vi "createPlatformDataV2.vi"() -> (3 "digital waveform":bool[](array[boolean]))   [LabVIEW 2017]
panel:
  in  "Platform 61":bool
  in  "Platform 60":bool
  in  "Platform 59":bool
  in  "Platform 58":bool
  in  "Platform 57":bool
  in  "Platform 56":bool
  in  "Platform 55":bool
  in  "Platform 54":bool
  in  "Platform 53":bool
  in  "Platform 52":bool
  in  "Platform 51":bool
  in  "Platform 50":bool
  in  "Platform 49":bool
  in  "Platform 48":bool
  in  "Platform 47":bool
  in  "Platform 46":bool
  in  "Platform 45":bool
  in  "Platform 44":bool
  in  "Platform 43":bool
  in  "Platform 42":bool
  in  "Platform 41":bool
  in  "Platform 40":bool
  in  "Platform 39":bool
  in  "Platform 38":bool
  in  "Platform 37":bool
  in  "Platform 36":bool
  in  "Platform 35":bool
  in  "Platform 34":bool
  in  "Platform 33":bool
  in  "Platform 32":bool
  in  "Platform 31":bool
  in  "Platform 30":bool
  in  "Platform 29":bool
  in  "Platform 28":bool
  in  "Platform 27":bool
  in  "Platform 26":bool
  in  "Platform 25":bool
  in  "Platform 24":bool
  in  "Platform 23":bool
  in  "Platform 22":bool
  in  "Platform 21":bool
  in  "Platform 20":bool
  in  "Platform 19":bool
  in  "Platform 18":bool
  in  "Platform 17":bool
  in  "Platform 16":bool
  in  "Platform 15":bool
  in  "Platform 14":bool
  in  "Platform 13":bool
  in  "Platform 12":bool
  in  "Platform 11":bool
  in  "Platform 10":bool
  in  "Platform 9":bool
  in  "Platform 8":bool
  in  "Platform 7":bool
  in  "Platform 6":bool
  in  "Platform 5":bool
  in  "Platform 4":bool
  in  "Platform 3":bool
  in  "Platform 2":bool
  in  "Platform 1":bool
  in  "Select?":bool
  in  "Platform 61":bool
  in  "Platform 60":bool
  in  "Platform 59":bool
  in  "Platform 58":bool
  in  "Platform 57":bool
  in  "Platform 56":bool
  in  "Platform 55":bool
  in  "Platform 54":bool
  in  "Platform 53":bool
  in  "Platform 52":bool
  in  "Platform 51":bool
  in  "Platform 50":bool
  in  "Platform 49":bool
  in  "Platform 48":bool
  in  "Platform 47":bool
  in  "Platform 46":bool
  in  "Platform 45":bool
  in  "Platform 44":bool
  in  "Platform 43":bool
  in  "Platform 42":bool
  in  "Platform 41":bool
  in  "Platform 40":bool
  in  "Platform 39":bool
  in  "Platform 38":bool
  in  "Platform 37":bool
  in  "Platform 36":bool
  in  "Platform 35":bool
  in  "Platform 34":bool
  in  "Platform 33":bool
  in  "Platform 32":bool
  in  "Platform 31":bool
  in  "Platform 30":bool
  in  "Platform 29":bool
  in  "Platform 28":bool
  in  "Platform 27":bool
  in  "Platform 26":bool
  in  "Platform 25":bool
  in  "Platform 24":bool
  in  "Platform 23":bool
  in  "Platform 22":bool
  in  "Platform 21":bool
  in  "Platform 20":bool
  in  "Platform 19":bool
  in  "Platform 18":bool
  in  "Platform 17":bool
  in  "Platform 16":bool
  in  "Platform 15":bool
  in  "Platform 14":bool
  in  "Platform 13":bool
  in  "Platform 12":bool
  in  "Platform 11":bool
  in  "Platform 10":bool
  in  "Platform 9":bool
  in  "Platform 8":bool
  in  "Platform 7":bool
  in  "Platform 6":bool
  in  "Platform 5":bool
  in  "Platform 4":bool
  in  "Platform 3":bool
  in  "Platform 2":bool
  in  "Platform 1":bool
  # "Platforms up"
  # "Platforms down"
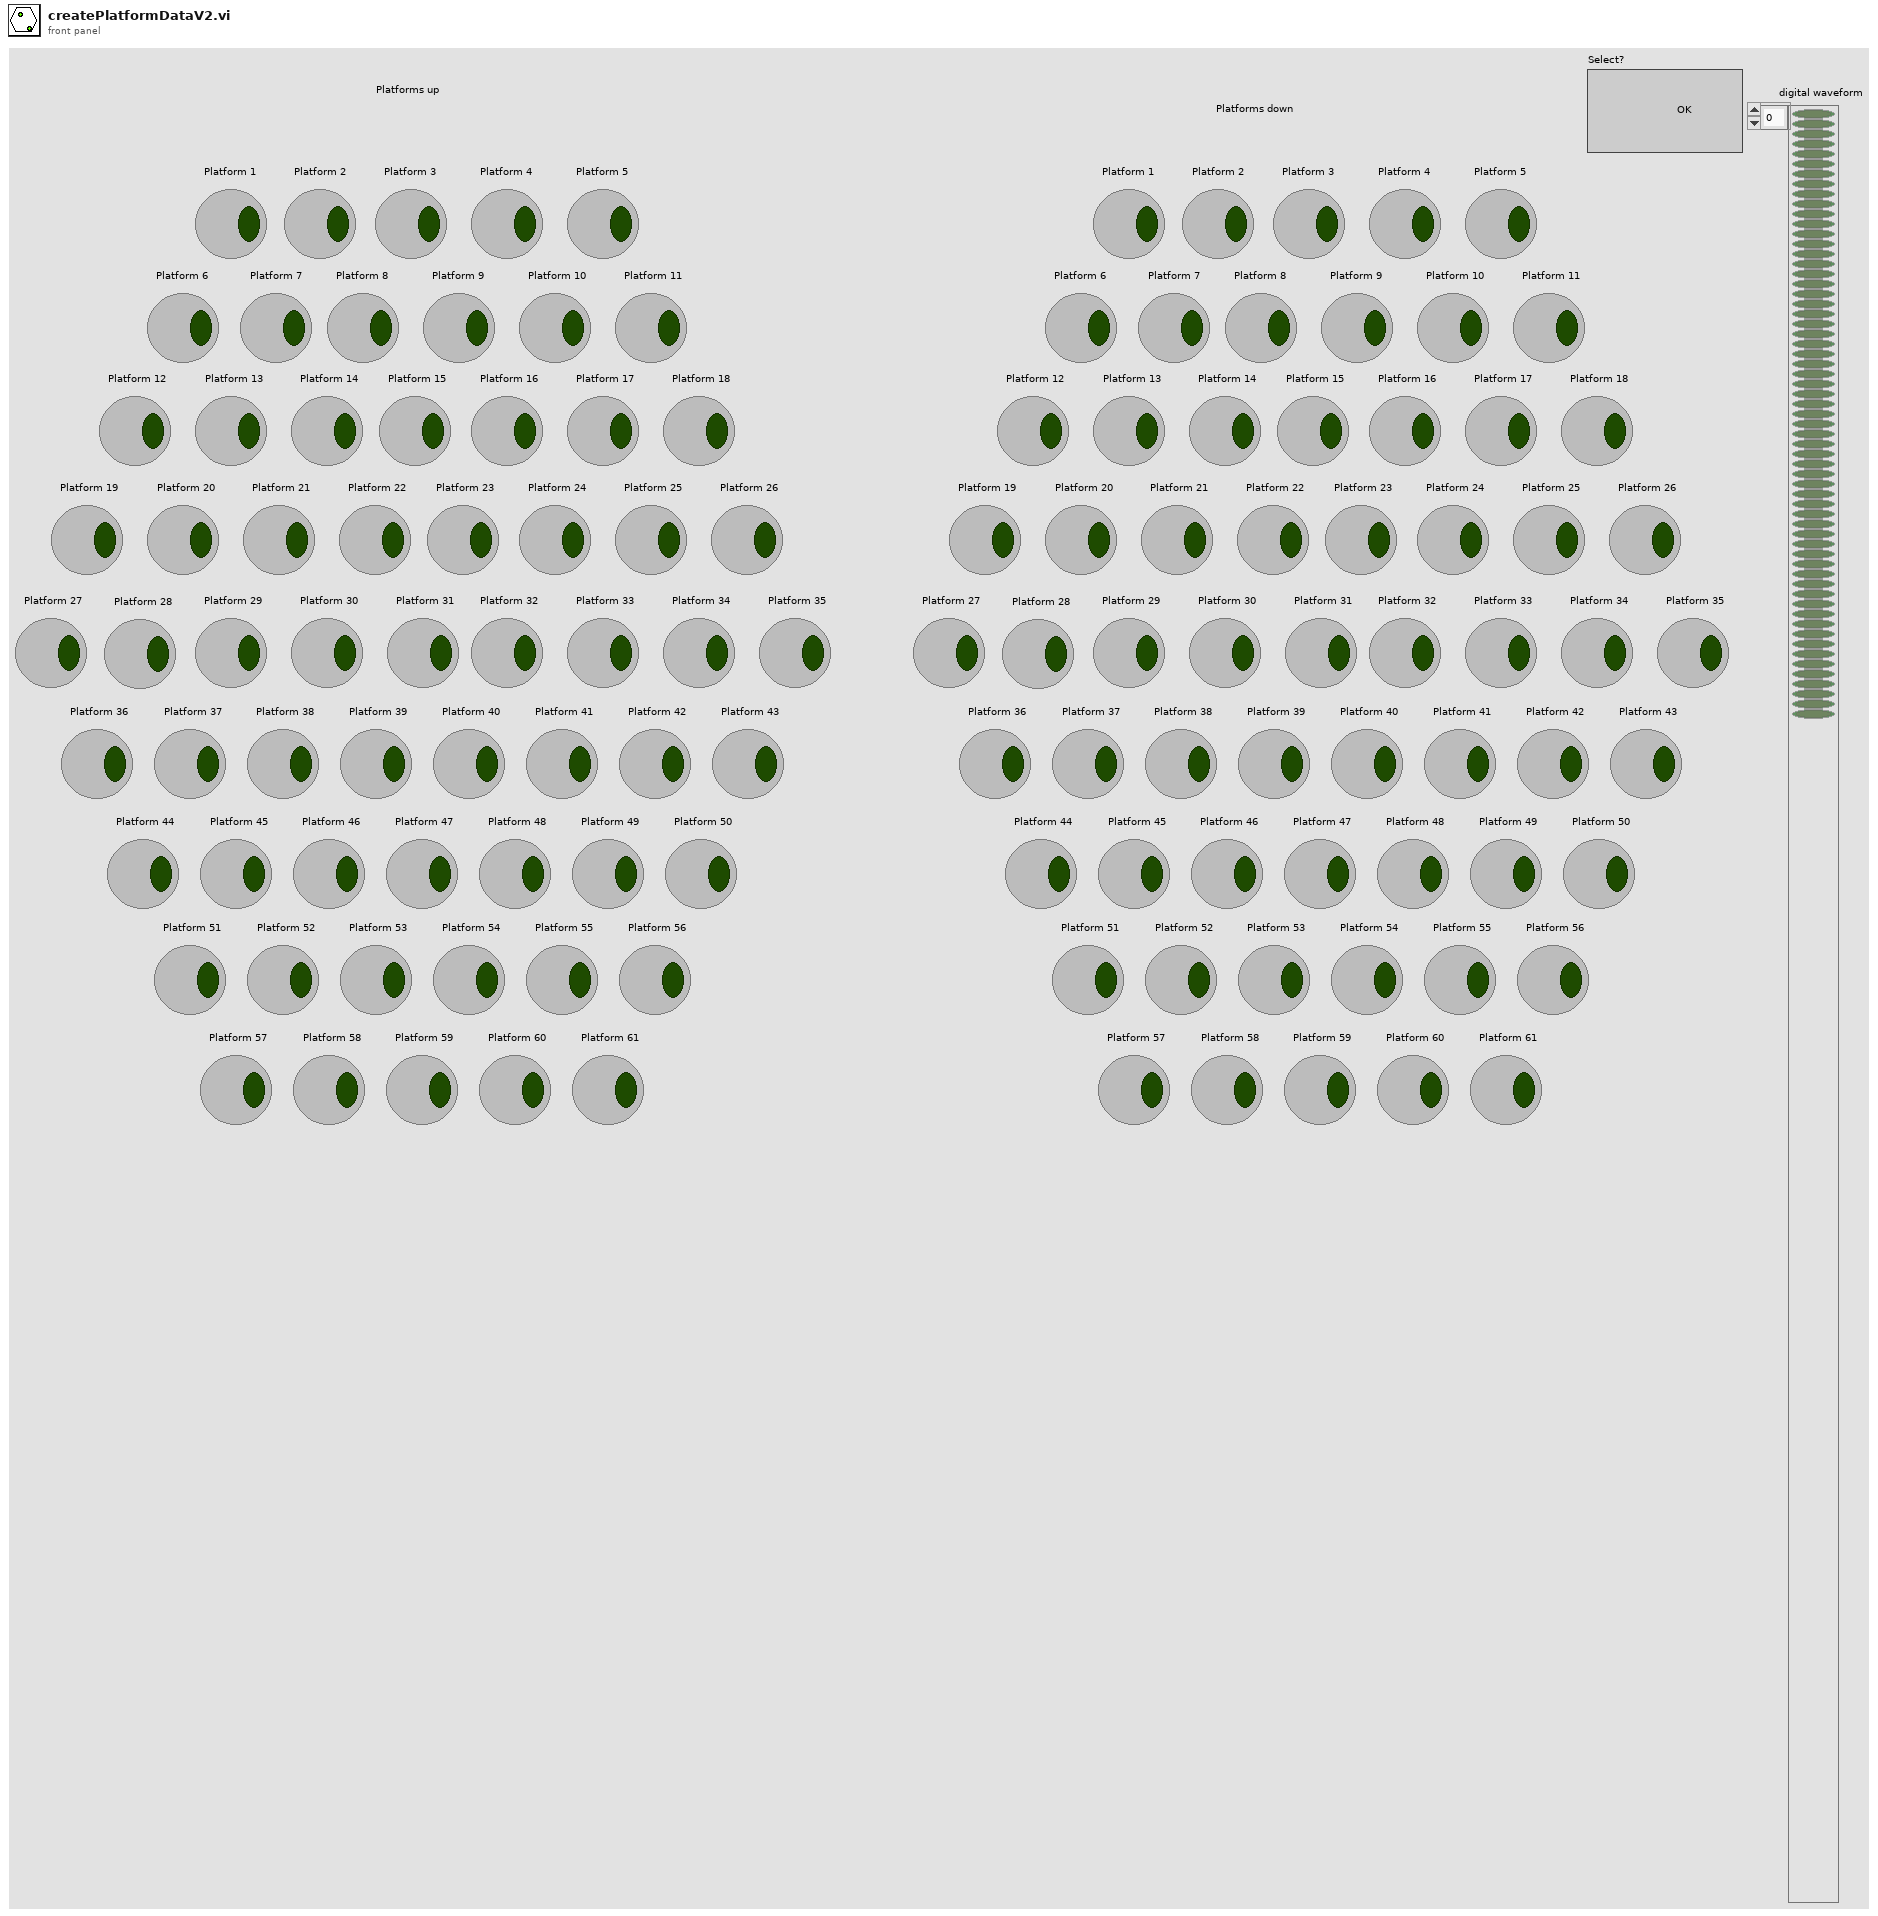
[diagram p1: front panel]
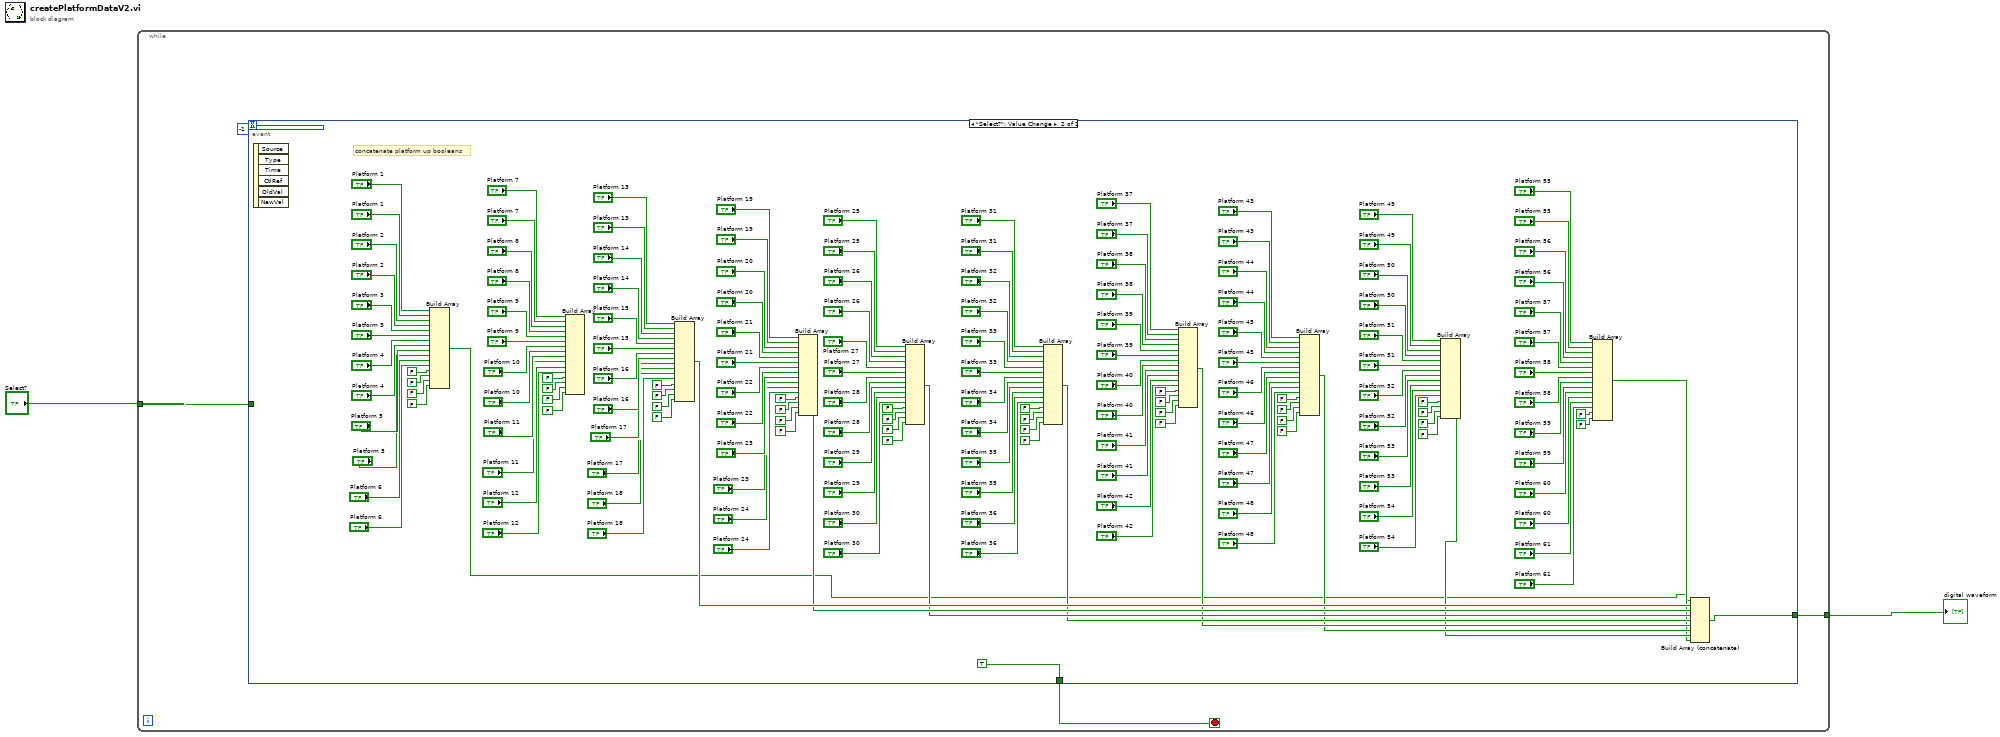
[diagram p0: block diagram]
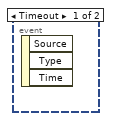
[diagram p2: hidden frame]
diagram:
  n1 = while {
    tunnel: "Select?" -> [w5]
    tunnel: [w3] -> w1
    stop <- w4 stop-if-true
    n2 = event shown="[1] \"Select?\": Value Change" {
      selector: _ -> [_ _]
      dyn-events: _ -> [_ _]
      timeout: -1 -> [_ _]
      tunnel: w5 -> [_ _]
      tunnel: [_ TRUE] -> w4
      tunnel: [_ w8] -> w3
      event Timeout {
        n3 = event-data() -> ()  [unwired: 1 in, 3 out]
      }
      event "Select?": Value Change {
        # "concatenate platform up booleans"
        n4 = event-data() -> ()  [unwired: 1 in, 6 out]
        n5 = Build Array("Platform 1", "Platform 1", "Platform 2", "Platform 2", "Platform 3", "Platform 3", "Platform 4", "Platform 4", "Platform 5", "Platform 5", "Platform 6", "Platform 6", FALSE, FALSE, FALSE, FALSE) -> (w7:bool[])
        n6 = Build Array("Platform 7", "Platform 7", "Platform 8", "Platform 8", "Platform 9", "Platform 9", "Platform 10", "Platform 10", "Platform 11", "Platform 11", "Platform 12", "Platform 12", FALSE, FALSE, FALSE, FALSE) -> ()  [unwired: 1 out]
        n7 = Build Array("Platform 13", "Platform 13", "Platform 14", "Platform 14", "Platform 15", "Platform 15", "Platform 16", "Platform 16", "Platform 17", "Platform 17", "Platform 18", "Platform 18", FALSE, FALSE, FALSE, FALSE) -> (w16:bool[])
        n8 = Build Array("Platform 19", "Platform 19", "Platform 20", "Platform 20", "Platform 21", "Platform 21", "Platform 22", "Platform 22", "Platform 23", "Platform 23", "Platform 24", "Platform 24", FALSE, FALSE, FALSE, FALSE) -> (w15:bool[])
        n9 = Build Array("Platform 25", "Platform 25", "Platform 26", "Platform 26", "Platform 27", "Platform 27", "Platform 28", "Platform 28", "Platform 29", "Platform 29", "Platform 30", "Platform 30", FALSE, FALSE, FALSE, FALSE) -> (w14:bool[])
        n10 = Build Array("Platform 31", "Platform 31", "Platform 32", "Platform 32", "Platform 33", "Platform 33", "Platform 34", "Platform 34", "Platform 35", "Platform 35", "Platform 36", "Platform 36", FALSE, FALSE, FALSE, FALSE) -> (w13:bool[])
        n11 = Build Array("Platform 37", "Platform 37", "Platform 38", "Platform 38", "Platform 39", "Platform 39", "Platform 40", "Platform 40", "Platform 41", "Platform 41", "Platform 42", "Platform 42", FALSE, FALSE, FALSE, FALSE) -> (w12:bool[])
        n12 = Build Array("Platform 43", "Platform 43", "Platform 44", "Platform 44", "Platform 45", "Platform 45", "Platform 46", "Platform 46", "Platform 47", "Platform 47", "Platform 48", "Platform 48", FALSE, FALSE, FALSE, FALSE) -> (w11:bool[])
        n13 = Build Array("Platform 49", "Platform 49", "Platform 50", "Platform 50", "Platform 51", "Platform 51", "Platform 52", "Platform 52", "Platform 53", "Platform 53", "Platform 54", "Platform 54", FALSE, FALSE, FALSE, FALSE) -> (w10:bool[])
        n14 = Build Array("Platform 55", "Platform 55", "Platform 56", "Platform 56", "Platform 57", "Platform 57", "Platform 58", "Platform 58", "Platform 59", "Platform 59", "Platform 60", "Platform 60", "Platform 61", "Platform 61", FALSE, FALSE) -> (w9:bool[])
        n15 = Build Array (concatenate)(w7, w16, w15, w14, w13, w12, w11, w10, w9) -> (w8:bool[])
      }
    }
  }
  "digital waveform" <- w1
